vi "WLAN - niVST - RFSG - ConfigureHW.vi"(0 "instrument handle":refnum<k15>, 11 "error in":errorcluster) -> (4 "instrument handle":refnum<k15>, 15 "error out":errorcluster)   [LabVIEW 2012]
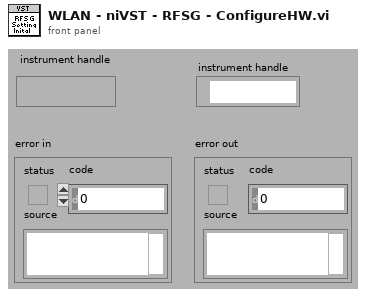
[diagram p1: front panel]
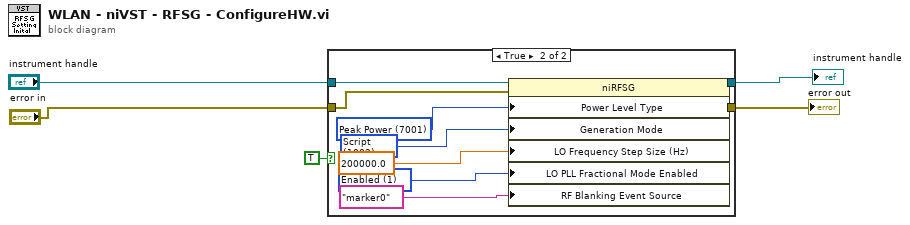
[diagram p0: block diagram]
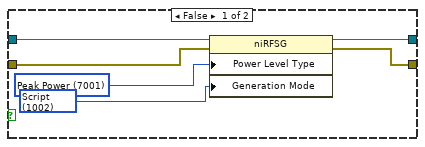
[diagram p2: hidden frame]
diagram:
  n1 = case shown="True" TRUE {
    tunnel: "error in" -> [w11 w20]
    tunnel: "instrument handle" -> [w10 w19]
    tunnel: [w7 w14] -> w5
    tunnel: [w6 w13] -> w1
    frame False {
      w9 = 7001 items=["Average Power"=7000, "Peak Power"=7001] ("RF:Power Level Type")
      w8 = 1002 items=["CW"=1000, "Arb Waveform"=1001, "Script"=1002] ("Arb:Generation Mode")
      n2 = property class="niRFSG"(reference=w10, error in=w11, "Power Level Type"=w9, "Generation Mode"=w8) -> (reference out=w6:refnum<k15>, error out=w7:errorcluster)
    }
    frame True {
      w15 = 1 items=["Disabled", "Enabled"] ("RF-RIO:Signal Path:LO PLL Fractional Mode Enabled (Hz)")
      w18 = 7001 items=["Average Power"=7000, "Peak Power"=7001] ("RF:Power Level Type")
      w17 = 1002 items=["CW"=1000, "Arb Waveform"=1001, "Script"=1002] ("Arb:Generation Mode")
      n3 = property class="niRFSG"(reference=w19, error in=w20, "Power Level Type"=w18, "Generation Mode"=w17, "LO Frequency Step Size (Hz)"=200000.0 ("RF-RIO:Signal Path:LO Frequency Step Size (Hz)"), "LO PLL Fractional Mode Enabled"=w15, "RF Blanking Event Source"="marker0" ("Device Specific:5644R and 5645R:Signal Path:RF Blanking Event Source")) -> (reference out=w13:refnum<k15>, error out=w14:errorcluster)
    }
  }
  "error out" <- w5
  "instrument handle" <- w1
